vi "Subscription Policy Initialize.vi"(8 "error in (no error)":errorcluster, 9 "Last Publish Time":timestamp, 10 "Last Topic Value":variant, 11 "OneShotSubscription In":refnum<class "OneShotSubscription.lvclass">) -> (0 "error out":errorcluster, 3 "OneShotSubscription Out":refnum<class "OneShotSubscription.lvclass">)   [LabVIEW 2015, in "Mediator.lvlib" / "OneShotSubscription.lvclass"]
uses:
  OneShotSubscription.lvclass
  OneShotSubscription.lvclass/OneShotSubscription.ctl
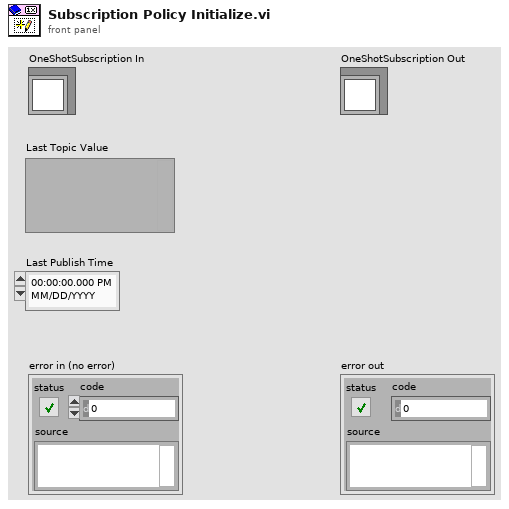
[diagram p1: front panel]
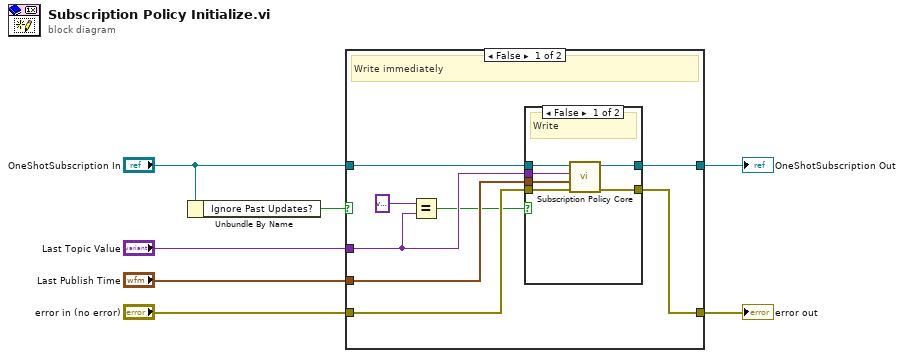
[diagram p0: block diagram]
diagram:
  n1 = Unbundle By Name("OneShotSubscription In") -> ("Ignore Past Updates?"=w5:bool)
  n2 = case shown="False" w5 {
    tunnel: "OneShotSubscription In" -> [w15 w25]
    tunnel: [w14 w25] -> w6
    tunnel: "Last Topic Value" -> [w10 _]
    tunnel: "Last Publish Time" -> [w12 _]
    tunnel: "error in (no error)" -> [w13 w24]
    tunnel: [w11 w24] -> w1
    frame False {
      # "Write immediately"
      n3 = Equal?(x=variant, y=w10) -> (x = y?=w8:bool)
      n4 = case shown="False" w8 {
        tunnel: w15 -> [w21 w23]
        tunnel: [w20 w23] -> w14
        tunnel: w13 -> [w19 w22]
        tunnel: w12 -> [w18 _]
        tunnel: [w17 w22] -> w11
        tunnel: w10 -> [w16 _]
        frame False {
          # "Write"
          n5 = call-dynamic "Subscription Policy Core.vi"("error in (no error)"=w19, "Publish Time"=w18, "New Topic Value"=w16, "OneShotSubscription In"=w21) -> ("error out"=w17:errorcluster, "OneShotSubscription Out"=w20:refnum<class "OneShotSubscription.lvclass">)  [unwired: 6 in]
        }
        frame True {
          # "Do not write\nimmediately\nif there is no\nvalue to write"
          # "No data yet"
        }
      }
    }
    frame True {
      # "Ignore past updates"
    }
  }
  "error out" <- w1
  "OneShotSubscription Out" <- w6
